vi "helper_checkForMonoBusy.vi"(8 "error in (no error)":errorcluster, 9 "milliseconds to wait":u32, 10 "Numeric":i32, 11 "Monochromator in":refnum<class "Monochromator.lvclass">) -> (0 "error out":errorcluster, 2 "iterations":i32, 3 "Monochromator out":refnum<class "Monochromator.lvclass">)   [LabVIEW 2023, in "horiba.test.lvlib"]
uses:
  horiba.test.lvlib
  Classes/Mono/Monochromator.lvclass
panel:
  # "Connector Pane"
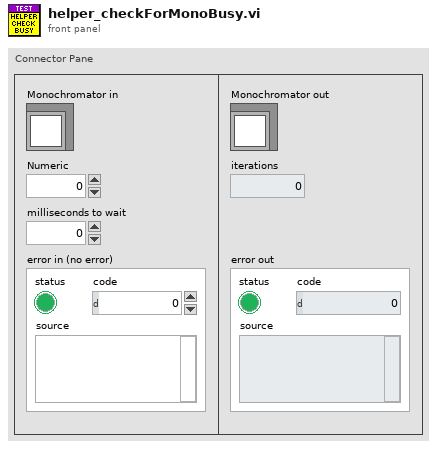
[diagram p1: front panel]
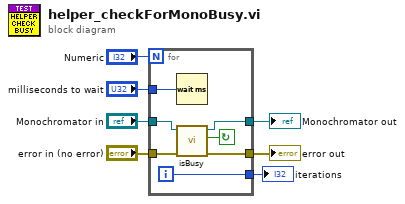
[diagram p0: block diagram]
diagram:
  n1 = for {
    N: "Numeric" -> [_]
    tunnel: "Monochromator in" -> [w14]
    tunnel: [w13] -> w5
    tunnel: "error in (no error)" -> [w12]
    tunnel: [w11] -> w6
    tunnel: "milliseconds to wait" -> [w9]
    tunnel: [w8] -> w1
    i -> [w8]
    stop <- w10 continue-if-true
    n2 = Wait (ms)(milliseconds to wait=w9) -> ()  [unwired: 1 out]
    n3 = call "isBusy.vi"("error in (no error)"=w12, "Monochromator in"=w14) -> ("error out"=w11:errorcluster, "mono is busy?"=w10:bool, "Monochromator out"=w13:refnum<class "Monochromator.lvclass">)  [unwired: 7 in]
  }
  "error out" <- w6
  "Monochromator out" <- w5
  "iterations" <- w1
